vi "0. Using within CSM - Get Module Configuration.vi"() -> ()   [LabVIEW 2017]
uses:
  fc5fbf42-5c4f-4ff1-85ec-327809f3c502.vi
  a48643ac-d5d5-4d55-bcec-da4c3fe174fc.vi
  08dfc535-f17e-4bcc-abdf-94a82fd10ea0.vi
  <userlib>/_NEVSTOP/Communicable State Machine(CSM)/AdvanceAPI/CSM - Revert Arguments-Safe String.vi
  <userlib>/_NEVSTOP/Communicable State Machine(CSM)/AdvanceAPI/CSM - Make String Arguments Safe.vi
  <userlib>/_NEVSTOP/Communicable State Machine(CSM)/AdvanceAPI/CSM - Break Down Multiple States String.vi
  <userlib>/_NEVSTOP/Communicable State Machine(CSM)/AdvanceAPI/CSM - Compact Multiple States.vi
  <userlib>/_NEVSTOP/Communicable State Machine(CSM)/AdvanceAPI/CSM - Keywords.vi
  <userlib>/_NEVSTOP/Communicable State Machine(CSM)/_Shared/Trim Single-line Text.vi
  addons/API-String-Arugments-Support/_Support/Query Data as API String Arguments(variant).vi
  addons/API-String-Arugments-Support/_Support/Convert API String Arguments to Data(variant).vi
  <userlib>/_NEVSTOP/Communicable State Machine(CSM)/Communicable State Machine.lvlib
  addons/API-String-Arugments-Support/API String Arguments Support.lvlib
panel:
  out "string":string
  out "bool":bool
  out "dbl":dbl
  out "cluster.string2":string
  out "cluster.bool2":bool
  out "State History":string
  out "Configurations":string[](array[string])
  out "VI Path":path
  out "Core.Current VI Reference":variant
  out "Core.Current VI Reference":string="DoA"
  out "Settings":string="DoA"
  out "error out":errorcluster
  out "DataBool":string="DoA"
  out "DataString":string="DoA"
  out "Settings.Bool":string="DoA"
  out "Settings.String":string="DoA"
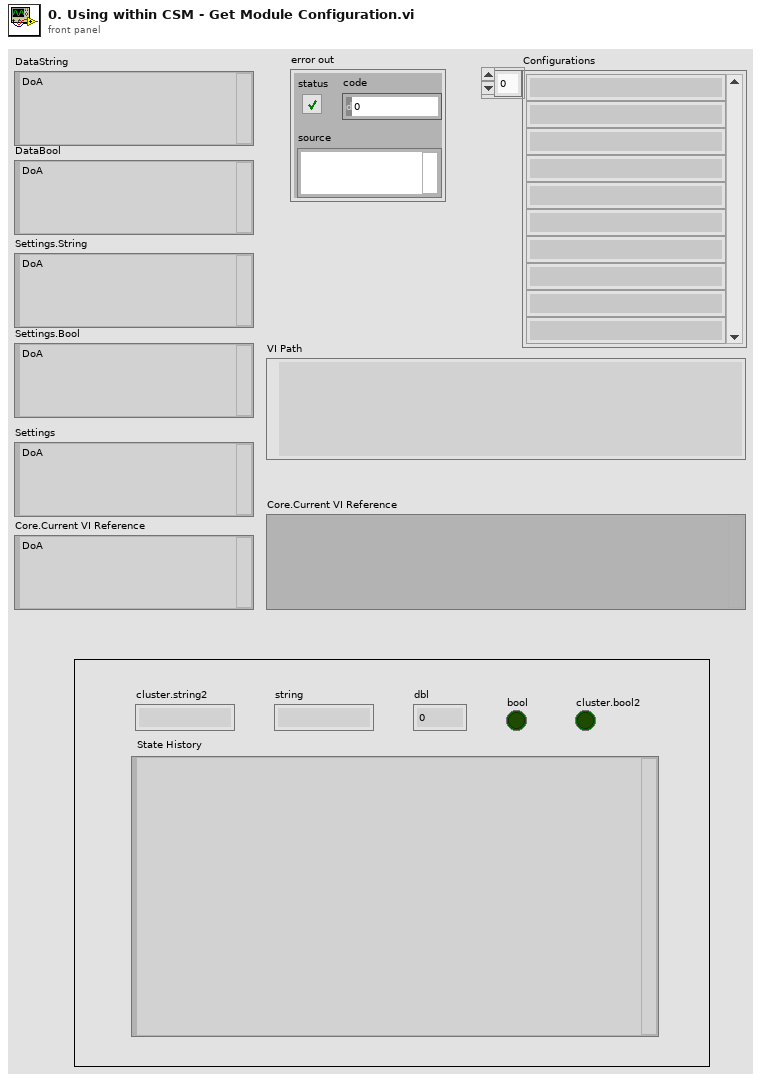
[diagram p1: front panel]
types:
  T1 = enum32{"Invalid", "Standard", "Closed", "Hidden", "Minimized", "Maximized"}
  T2 = enum32{"invalid app kind", "Development System", "Run Time System", "Student Edition", "Embedded LabVIEW", "Evaluation", "Custom"}
  T3 = typedef "Communicable State Machine.lvlib/_CSM_Response Source Message.ctl" = cluster{"‘State":string, "’Arguments":string, "’Error":errorcluster}
  T4 = cluster{"Current VI Reference":refnum<vi>, "Close Panel on Exit?":bool}
  T5 = cluster{"Core":cluster{"Current VI Reference":refnum<vi>, "Close Panel on Exit?":bool}, "DataBool":bool, "DataString":string, "Settings":cluster{"Bool":bool, "string":string}}
  T6 = cluster{"string":string, "bool":bool, "dbl":dbl, "cluster":cluster{"string2":string, "bool2":bool}}
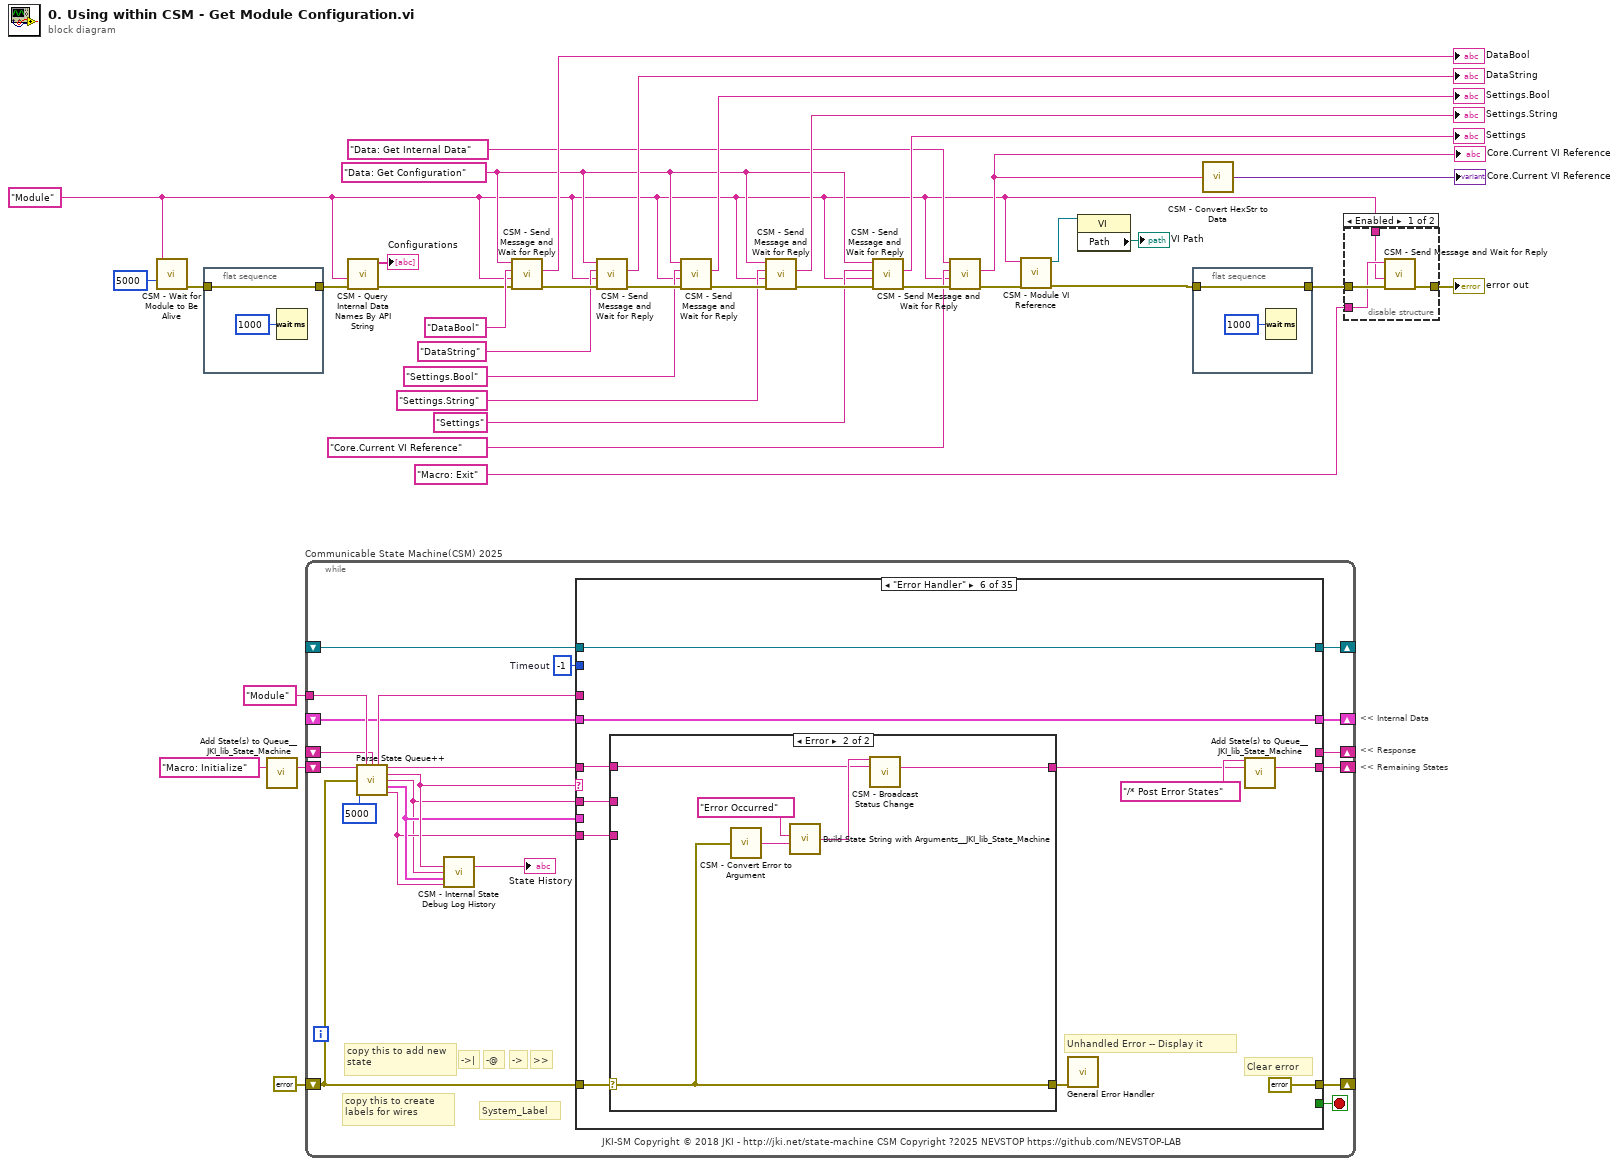
[diagram p0: block diagram]
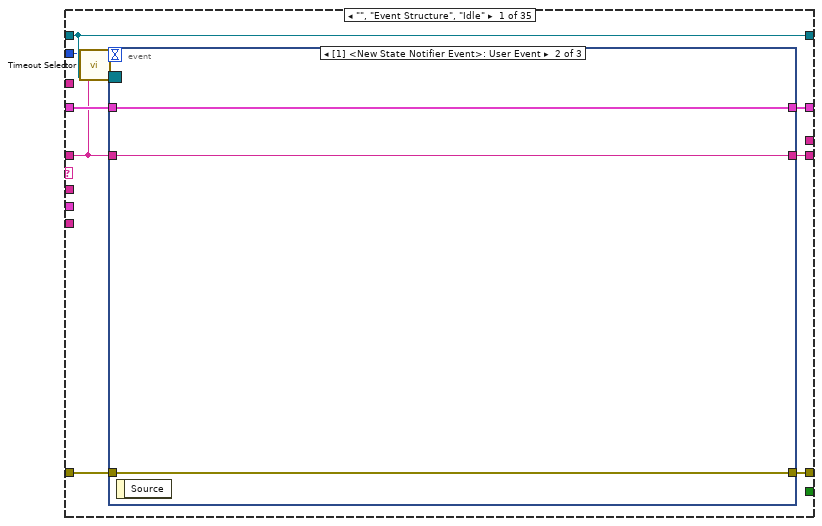
[diagram p2: hidden frame]
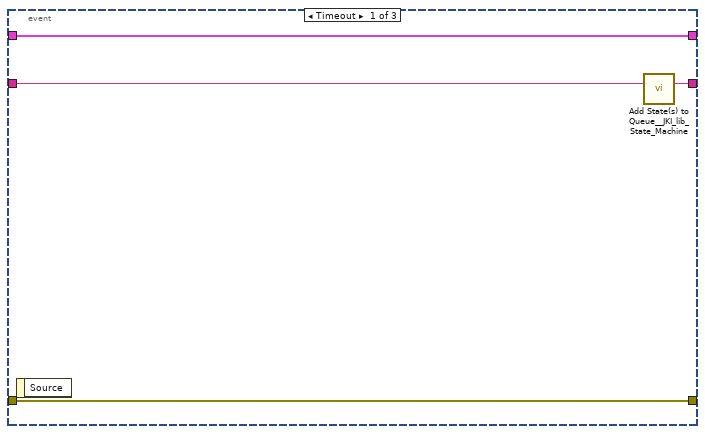
[diagram p3: hidden frame]
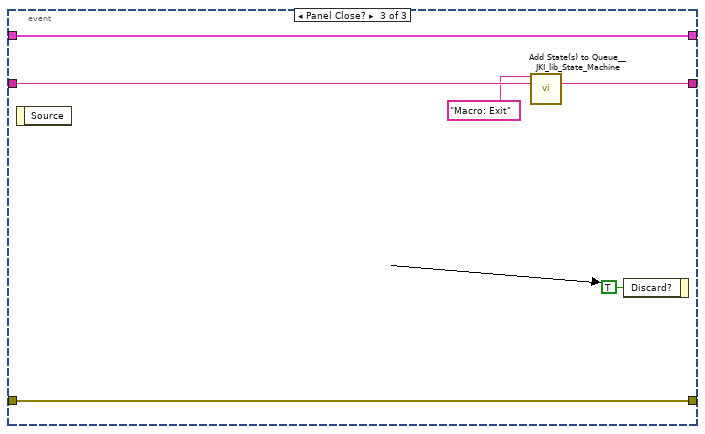
[diagram p4: hidden frame]
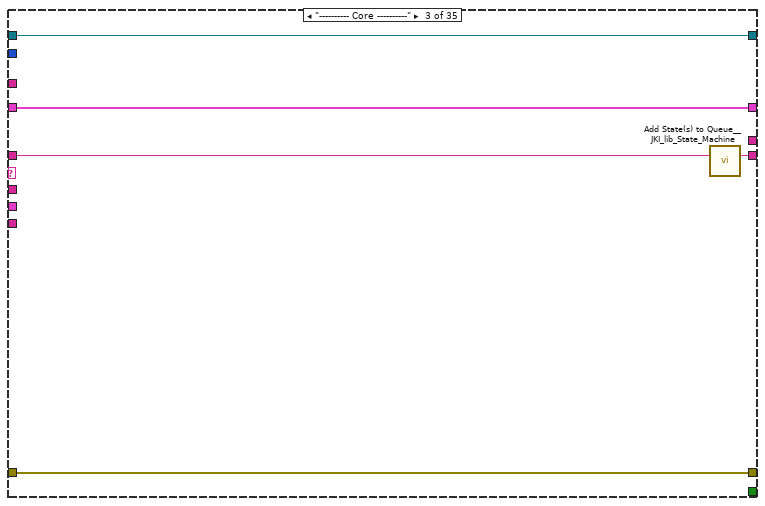
[diagram p6: hidden frame]
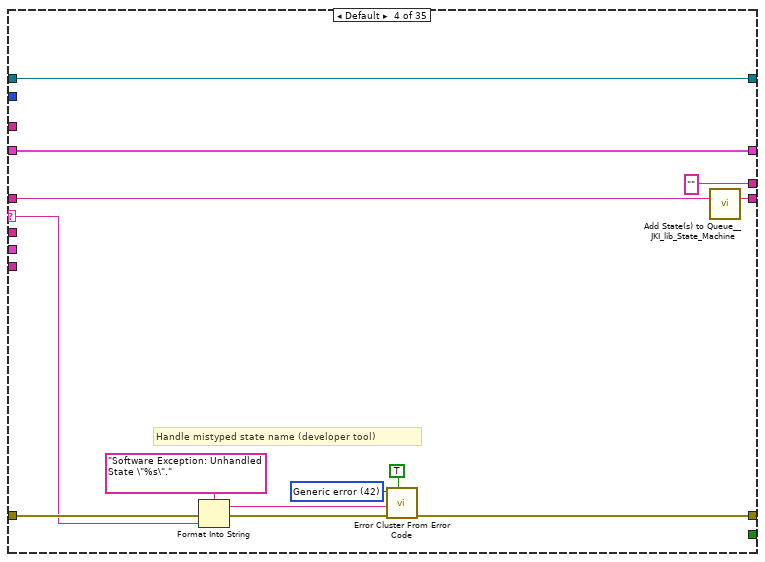
[diagram p7: hidden frame]
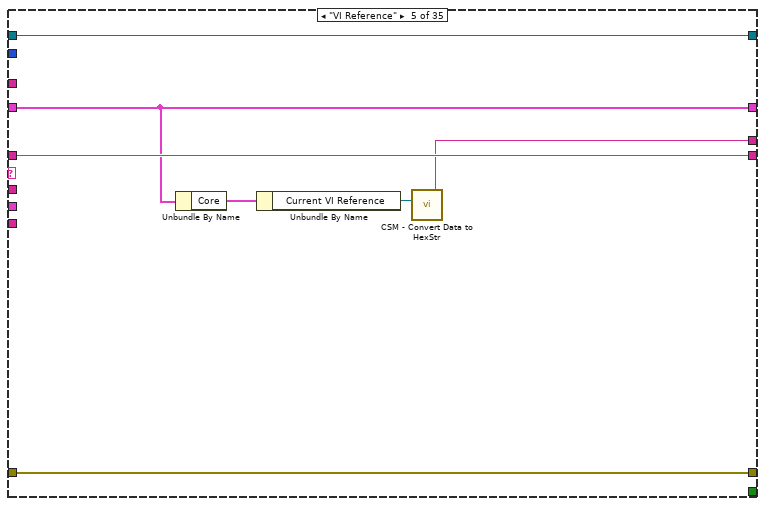
[diagram p8: hidden frame]
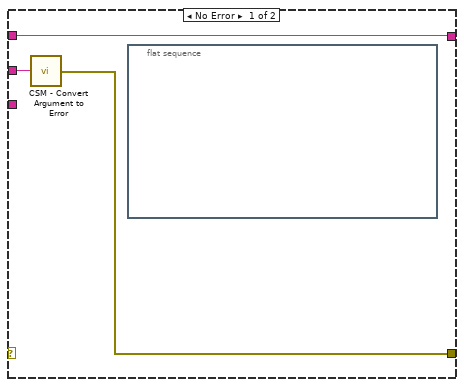
[diagram p9: hidden frame]
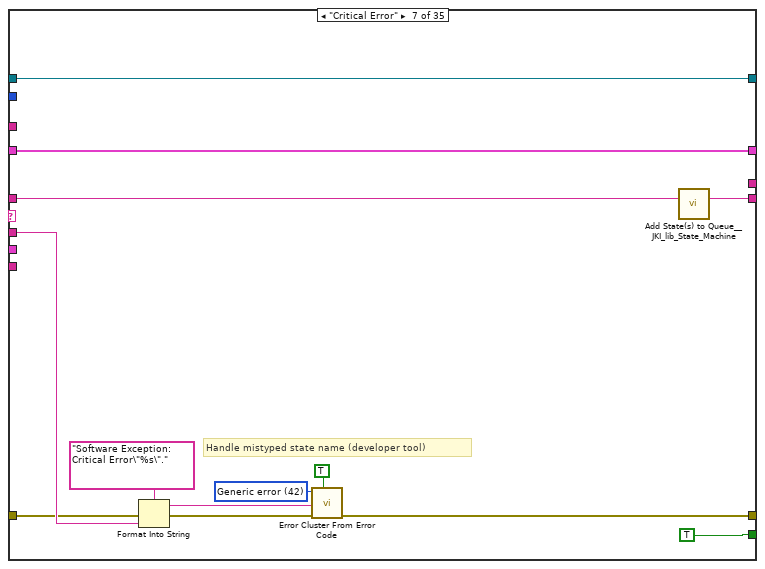
[diagram p10: hidden frame]
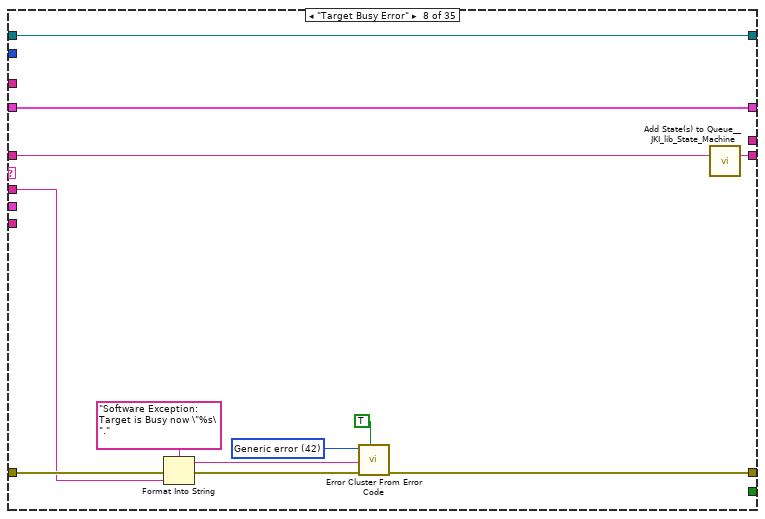
[diagram p11: hidden frame]
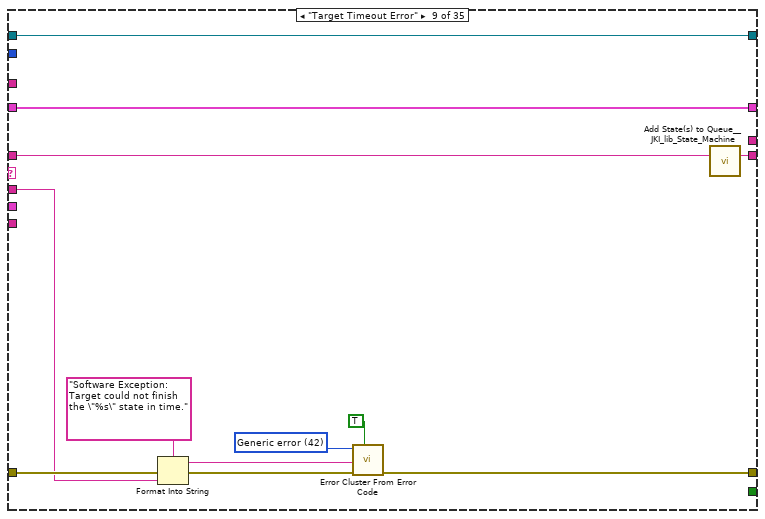
[diagram p12: hidden frame]
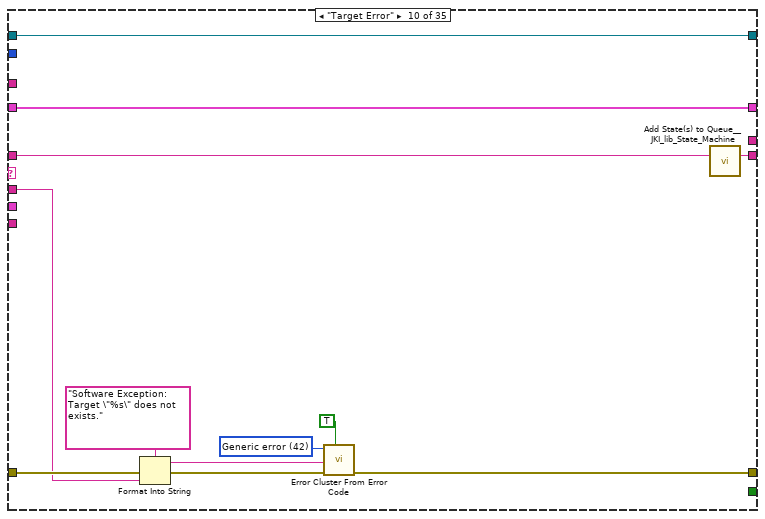
[diagram p13: hidden frame]
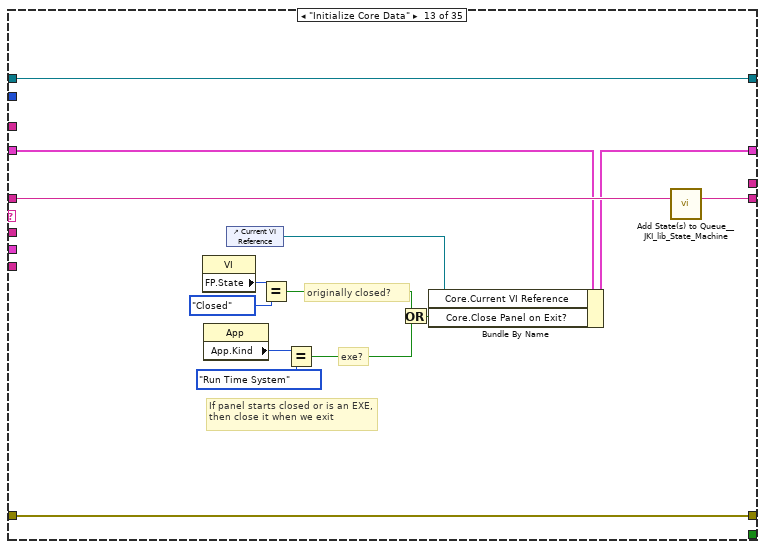
[diagram p16: hidden frame]
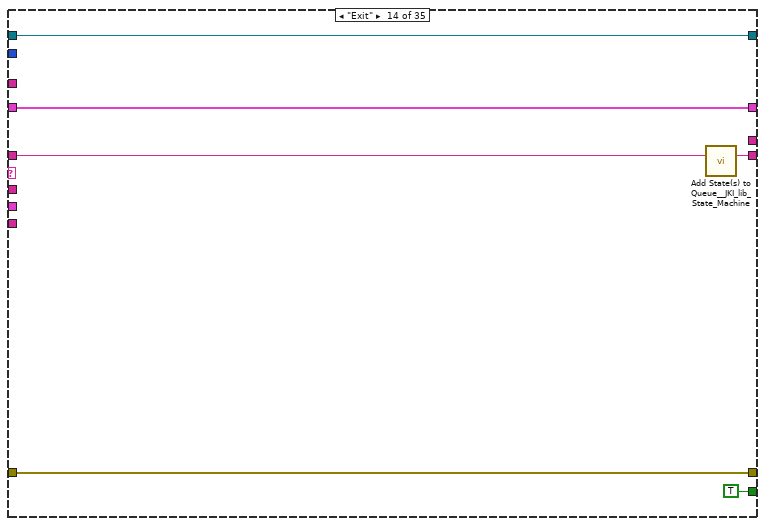
[diagram p17: hidden frame]
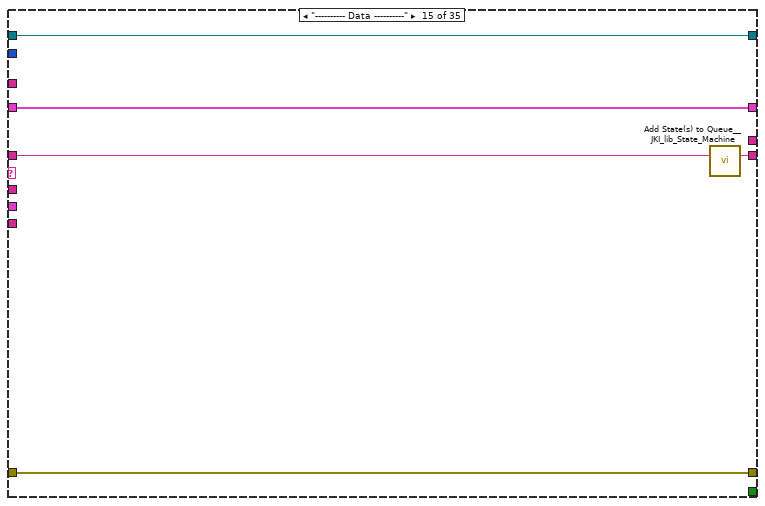
[diagram p18: hidden frame]
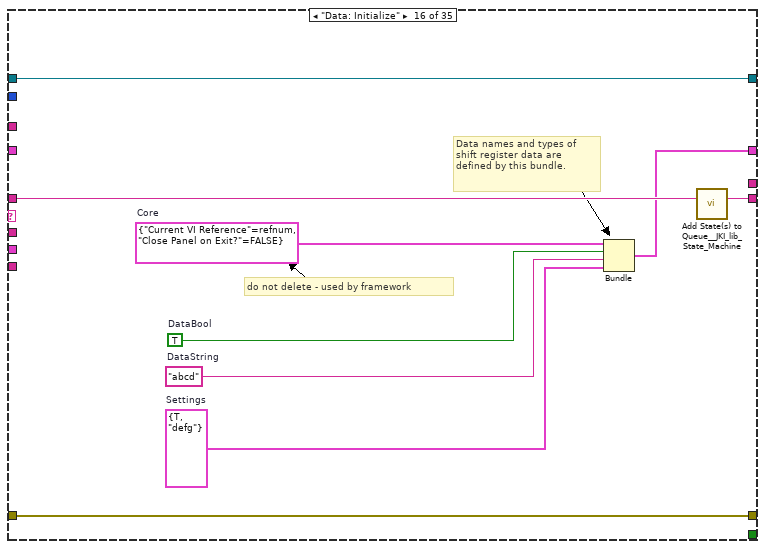
[diagram p19: hidden frame]
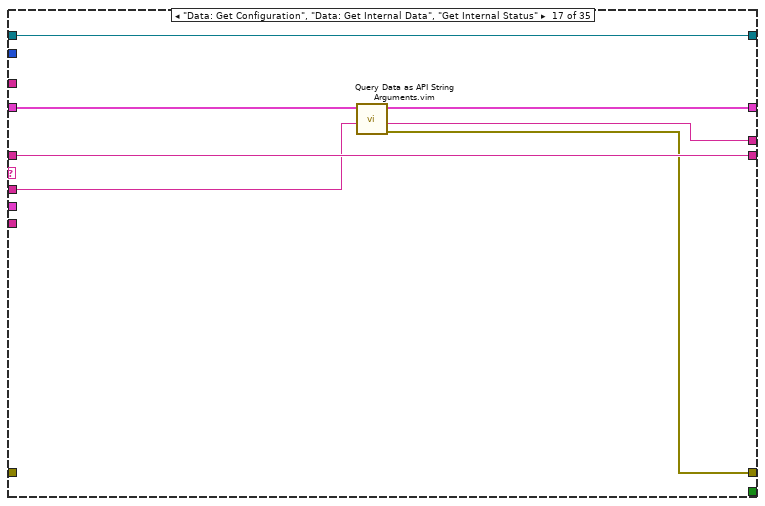
[diagram p20: hidden frame]
diagram:
  w22 = "Data: Get Configuration" ("Name(\"\" to use uuid)")
  w5 = "Module" ("Name(\"\" to use uuid)")
  # "<< Internal Data"
  # "<< Response"
  # "<< Remaining States"
  n1 = call <userlib>:"CSM - Wait for Module to Be Alive.vi"("CSM Name"=w5, "Wait (5000 ms)"=5000 ("Wait(5000ms)")) -> ("error out"=w7:errorcluster)  [unwired: 11 in, 2 out]
  n2 = flat-sequence {
    tunnel: [w39] -> w10
    tunnel: w7 -> [w39]
    frame #0 {
      n3 = Wait (ms)(milliseconds to wait=u32 1000) -> ()  [unwired: 1 out]
    }
  }
  n4 = call <vilib>:"Add State(s) to Queue__JKI_lib_State_Machine.vi"("State(s) in (\"\")"="Macro: Initialize") -> ("States Out"=w2:string)  [unwired: 14 in]
  n5 = while "Communicable State Machine(CSM) 2025" {
    shift-right: [w55] -> _
    shift-left: _ -> [w41]
    shift-right: [w58] -> _
    shift-left: errorcluster {"status"=FALSE, "code"=0, "source"=""} ("error") -> [w53]
    shift-right: [w57] -> _
    shift-left: w2 -> [w59]
    tunnel: "Module" ("Name(\"\" to use uuid)") -> [w48]
    shift-right: [w51] -> _
    shift-left: _ -> [w43]
    shift-right: [w50] -> _
    shift-left: _ -> [w49]
    stop <- w56 stop-if-true
    w54 = -1  # Timeout
    # "JKI-SM Copyright © 2018 JKI - http://jki.net/state-machine CSM Copyright ?2025 NEVSTOP https://github.com/NEVSTOP-LAB"
    # "->|"
    # "copy this to add new state"
    # ">>"
    # "->"
    # "-@"
    # "copy this to create labels for wires"
    # "System_Label"
    n6 = call <userlib>:"Parse State Queue++.vi"("State Queue"=w59, "Name (\"\" to Use UUID)"=w48, "Response Arguments"=w43, "Previous Error"=w53, "Response Timeout (-2 Use Global Settings)"=5000 ("Response Timeout(1000ms)")) -> ("Name Used"=w44:string, "Remaining States"=w60:string, "Current State"=w47:string, "Arguments"=w42:string, "Additional Information"=w46:T3, "Source CSM"=w45:string)  [unwired: 5 in]
    n7 = call <userlib>:"CSM - Internal State Debug Log History.vi"("State"=w47, "Arguments (\"\")"=w42, ">> Response Source Message >>"=w46, "Source (\"\")"=w45) -> ("Debug Log"=→"State History":string)  [unwired: 11 in]
    n8 = case shown="\"Error Handler\"" w47 {
      selector: w47 -> [_ _ _ w94 _ _ _ _ _ _ _ _ _ _ _ _ _ _ _ _ _ _ _ _ _ _ _ _ _ _ _ _ _ _ _]
      tunnel: w60 -> [w61 w86 w91 w98 w110 w115 w143 w146 w163 w175 w183 w187 w202 w208 w213 w222 w229 w235 w242 w247 w254 w258 w264 w269 w276 w292 w362 w368 w379 w382 w395 w398 w404 w409 w414]
      tunnel: w42 -> [_ _ _ _ _ w113 w136 w148 w159 w171 _ _ _ _ _ _ w224 w233 _ _ _ _ _ _ w271 w286 _ _ _ _ w391 _ _ _ _]
      tunnel: w41 -> [w68 w85 w88 w96 w106 w121 w144 w150 w161 w173 w182 w186 w195 w206 w210 _ w227 w232 w237 w244 w253 w257 w261 w267 w274 w288 w359 w365 w376 w381 w394 w397 w401 w406 w411]
      tunnel: [w67 w84 w89 w100 w111 errorcluster {"status"=FALSE, "code"=0, "source"=""} ("error out") w132 w145 w157 w169 w184 w188 w199 w205 w211 w219 w225 w230 w238 w245 w248 w256 w262 w266 w272 w289 w360 w366 w377 w383 w384 w399 w402 w407 w412] -> w58
      tunnel: w53 -> [w66 w84 w89 w99 w111 w119 w133 w152 w164 w176 w184 w188 w199 w205 w211 w219 _ _ w239 w245 _ w259 w262 w266 w273 w290 w360 w366 w377 w383 _ w399 w402 w407 w412]
      tunnel: [w69 w86 w90 w97 w110 w117 w142 w151 w162 w174 w183 w187 w201 w207 w212 w221 w229 w235 w241 w246 w254 w258 w263 w268 w275 w291 w361 w367 w378 w382 w395 w398 w403 w408 w413] -> w57
      tunnel: [_ _ _ _ _ _ TRUE _ _ _ _ _ _ TRUE _ _ _ _ _ _ _ _ _ _ _ _ _ _ _ _ _ _ _ _ _] -> w56
      tunnel: [w65 w85 w88 w96 w106 w121 w144 w150 w161 w173 w182 w186 w200 w206 w210 w220 w223 w231 w237 w244 w253 w257 w261 w267 w274 w288 w359 w365 w376 w381 w394 w397 w401 w406 w411] -> w55
      tunnel: w54 -> [w63 _ _ _ _ _ _ _ _ _ _ _ _ _ _ _ _ _ _ _ _ _ _ _ _ _ _ _ _ _ _ _ _ _ _]
      tunnel: w45 -> [_ _ _ _ _ w112 _ _ _ _ _ _ _ _ _ _ _ _ _ _ _ _ _ _ _ _ _ _ _ _ _ _ _ _ _]
      tunnel: w46 -> [_ _ _ _ _ _ _ _ _ _ _ _ _ _ _ _ _ _ _ _ _ _ _ _ _ _ _ _ _ _ _ _ _ _ _]
      tunnel: [_ _ _ "" w105 _ _ _ _ _ _ _ _ _ _ _ w226 _ _ _ _ _ _ _ _ _ _ _ _ _ _ _ _ _ _] -> w51
      tunnel: [w64 w83 w87 w92 w109 w120 w134 w147 w158 w170 w181 w185 w189 w203 w209 w215 w228 w234 w236 w243 w252 w255 w260 w265 w270 w285 w358 w363 w369 w380 w393 w396 w400 w405 w410] -> w50
      tunnel: w49 -> [w64 w83 w87 w92 w109 w120 w134 w147 w158 w170 w181 w185 w189 w203 w209 w215 w228 w234 w236 w243 _ w255 w260 w265 w270 w285 w358 w363 w369 w380 w393 w396 w400 w405 w410]
      tunnel: w44 -> [_ _ _ _ _ _ _ _ _ _ _ _ _ _ _ _ _ _ _ _ w251 _ _ _ _ _ _ _ _ _ _ _ _ _ _]
      frame "", "Event Structure", "Idle" {
        n9 = call <userlib>:"Timeout Selector.vi"("Remaining States"=w61, "Timeout Expected"=w63) -> ("Timeout"=w62:i32)  [unwired: 5 in]
        n10 = event shown="[1] <New State Notifier Event>: User Event" {
          selector: w64 -> [_ _ _]
          dyn-events: _ -> [_ _ _]
          timeout: w62 -> [_ _ _]
          tunnel: w61 -> [w73 w75 w82]
          tunnel: [w72 w75 w81] -> w69
          tunnel: w68 -> [w70 w76 w79]
          tunnel: [w71 w74 w80] -> w67
          tunnel: w66 -> [w71 w74 w80]
          tunnel: [w70 w76 w79] -> w65
          event Timeout {
            n11 = event-data() -> ()  [unwired: 1 in, 1 out]
            n12 = call <vilib>:"Add State(s) to Queue__JKI_lib_State_Machine.vi"("State(s) in (\"\")"=w73) -> ("States Out"=w72:string)  [unwired: 14 in]
          }
          event User Event {
            n13 = event-data() -> ()  [unwired: 1 in, 1 out]
          }
          event Panel Close? {
            n14 = event-data() -> ()  [unwired: 1 in, 1 out]
            n15 = call <vilib>:"Add State(s) to Queue__JKI_lib_State_Machine.vi"("State(s) in Front (\"\")"="Macro: Exit", "State(s) in (\"\")"=w82) -> ("States Out"=w81:string)  [unwired: 13 in]
            n16 = event-data("Discard?"=TRUE) -> ()  [unwired: 1 in, 1 out]
          }
        }
      }
      frame "CSM Documentation" {
        # "CSM Documentation"
      }
      frame "---------- Core ----------" {
        n17 = call <vilib>:"Add State(s) to Queue__JKI_lib_State_Machine.vi"("State(s) in (\"\")"=w91) -> ("States Out"=w90:string)  [unwired: 14 in]
      }
      frame Default {
        w103 = 42 items=["No error", "Argument error", "Memory is full", "Out of zone", "End of file", "File already open", "Generic file I/O error", "File not found", "File permission error", "Disk is full", "Duplicate path", "Too many files open", "System feature not enabled", "Resource file not found", "Cannot add resource", "Resource not found", "Image not found", "Image memory error", "Pen does not exist", "Config type invalid", "Config token not found", "Config parse error", "Config memory error", "Bad external code format", "Bad external code offset", "External code not present", "Null window", "Destroy window error", "Null menu", "Print aborted", "Bad print record", "Print driver error", "Windows error during printing", "Memory error during printing", "Print dialog error", "Generic print error", "Invalid device refnum", "Device not found", "Device parameter error", "Device unit error", "Cannot open device", "Device call aborted", "Generic error", "Cancelled by user", "Object ID too low", "Object ID too high", "Object not in heap", "Unknown heap", "Unknown object (invalid DefProc)", "Unknown object (DefProc not in table)", "Message out of range", "Invalid (null) method", "Unknown message", "Manager call not supported", "Bad address", "Network operation in progress", "Network operation timed out", "Connection is busy", "Network attribute not supported", "Network error", "Address in use", "System out of memory", "Connection aborted", "Connection refused", "Not connected", "Already connected", "Connection closed", "Initialization error (interapplication manager)", "Bad occurrence", "Wait on unbound occurrence handler", "Occurrence queue overflow", "Datalog type conflict", "Unused", "Unrecognized type (interapplication manager)", "Memory corrupt", "Failed to make temporary DLL", "Old CIN version", "Drag socket not found", "Failed to load drop-object", "Failed to register OLE object", "Failed to release OLE object", "Format specifier type mismatch", "Unknown format specifier", "Too few format specifiers", "Too many format specifiers", "Scan failed", "Newer CIN version", "Error converting to variant", "Runtime menu error", "Password tampered", "Variant attribute not found", "Incompatible variant data type", "Event data is not available", "Event Store is not present", "Occurrence is not found", "Event Queue is not created", "Event info is not available", "Refnum passed is NULL", "Error retrieving Class GUID", "Error retrieving CoClass GUID", "Error retrieving TypeLib GUID.", "Bad built application magic bytes.", "Specific driver is different from the specific driver associated with the Logical Name.", "There is no session opened to the class driver.", "Max Error", "MAX - Error with config objects", "MAX - Error loading configuration", "MAX - Group not supported"]
        # "Handle mistyped state name (developer tool)"
        n18 = Format Into String(format string="Software Exception: Unhandled State \"%s\"." ("message"), error in=w99, w94) -> (resulting string=w102:string, error out=w101:errorcluster)  [unwired: 1 in]
        n19 = call <vilib>:"Error Cluster From Error Code.vi"("show call chain? (False)"=TRUE, "error in (no error)"=w101, "error message (\"\")"=w102, "error code (0)"=w103) -> ("error out"=w100:errorcluster)  [unwired: 5 in]
        n20 = call <vilib>:"Add State(s) to Queue__JKI_lib_State_Machine.vi"("State(s) in (\"\")"=w98) -> ("States Out"=w97:string)  [unwired: 14 in]
      }
      frame "VI Reference" {
        n21 = Unbundle By Name(w106) -> ("Core"=w108:T4)
        n22 = Unbundle By Name(w108) -> ("Current VI Reference"=w107:refnum<vi>)
        n23 = call <userlib>:"CSM - Convert Data to HexStr.vi"("Variant"=w107) -> ("HEX String (0-9,A-F)"=w105:string)  [unwired: 8 in]
      }
      frame "Error Handler" {
        # "Unhandled Error -- Display it"
        # "Clear error"
        n24 = case shown="Error" w119 {
          selector: w119 -> [_ w126]
          tunnel: [w124 w128] -> w116
          tunnel: w115 -> [w124 w127]
          tunnel: [w123 w126] -> w114
          tunnel: w113 -> [w125 _]
          tunnel: w112 -> [_ _]
          frame No Error {
            n25 = call <userlib>:"CSM - Convert Argument to Error.vi"("Argument"=w125) -> ("Error"=w123:errorcluster)  [unwired: 4 in]
            n26 = flat-sequence {
              frame #0 {
              }
            }
          }
          frame Error {
            n27 = call <userlib>:"CSM - Convert Error to Argument.vi"("Error"=w126) -> ("Argument"=w130:string)  [unwired: 4 in]
            n28 = call <vilib>:"Build State String with Arguments__JKI_lib_State_Machine.vi"("Arguments (\"\")"=w130, "State"="Error Occurred" ("Status with Arguments")) -> ("State with Arguments"=w129:string)  [unwired: 4 in]
            n29 = call <userlib>:"CSM - Broadcast Status Change.vi"("Status With Arguments"=w129, "State Queue"=w127) -> ("Remaining States"=w128:string)  [unwired: 13 in]
          }
        }
        n30 = call <vilib>:"General Error Handler.vi"("error in (no error)"=w114) -> ()  [unwired: 10 in, 5 out]
        n31 = call <vilib>:"Add State(s) to Queue__JKI_lib_State_Machine.vi"("State(s) in Front (\"\")"="/* Post Error States", "State(s) in (\"\")"=w116) -> ("States Out"=w117:string)  [unwired: 13 in]
      }
      frame "Critical Error" {
        w140 = 42 items=["No error", "Argument error", "Memory is full", "Out of zone", "End of file", "File already open", "Generic file I/O error", "File not found", "File permission error", "Disk is full", "Duplicate path", "Too many files open", "System feature not enabled", "Resource file not found", "Cannot add resource", "Resource not found", "Image not found", "Image memory error", "Pen does not exist", "Config type invalid", "Config token not found", "Config parse error", "Config memory error", "Bad external code format", "Bad external code offset", "External code not present", "Null window", "Destroy window error", "Null menu", "Print aborted", "Bad print record", "Print driver error", "Windows error during printing", "Memory error during printing", "Print dialog error", "Generic print error", "Invalid device refnum", "Device not found", "Device parameter error", "Device unit error", "Cannot open device", "Device call aborted", "Generic error", "Cancelled by user", "Object ID too low", "Object ID too high", "Object not in heap", "Unknown heap", "Unknown object (invalid DefProc)", "Unknown object (DefProc not in table)", "Message out of range", "Invalid (null) method", "Unknown message", "Manager call not supported", "Bad address", "Network operation in progress", "Network operation timed out", "Connection is busy", "Network attribute not supported", "Network error", "Address in use", "System out of memory", "Connection aborted", "Connection refused", "Not connected", "Already connected", "Connection closed", "Initialization error (interapplication manager)", "Bad occurrence", "Wait on unbound occurrence handler", "Occurrence queue overflow", "Datalog type conflict", "Unused", "Unrecognized type (interapplication manager)", "Memory corrupt", "Failed to make temporary DLL", "Old CIN version", "Drag socket not found", "Failed to load drop-object", "Failed to register OLE object", "Failed to release OLE object", "Format specifier type mismatch", "Unknown format specifier", "Too few format specifiers", "Too many format specifiers", "Scan failed", "Newer CIN version", "Error converting to variant", "Runtime menu error", "Password tampered", "Variant attribute not found", "Incompatible variant data type", "Event data is not available", "Event Store is not present", "Occurrence is not found", "Event Queue is not created", "Event info is not available", "Refnum passed is NULL", "Error retrieving Class GUID", "Error retrieving CoClass GUID", "Error retrieving TypeLib GUID.", "Bad built application magic bytes.", "Specific driver is different from the specific driver associated with the Logical Name.", "There is no session opened to the class driver.", "Max Error", "MAX - Error with config objects", "MAX - Error loading configuration", "MAX - Group not supported"]
        # "Handle mistyped state name (developer tool)"
        n32 = Format Into String(format string="Software Exception: Critical Error\"%s\"." ("message"), error in=w133, w136) -> (resulting string=w139:string, error out=w138:errorcluster)  [unwired: 1 in]
        n33 = call <vilib>:"Error Cluster From Error Code.vi"("show call chain? (False)"=TRUE, "error in (no error)"=w138, "error message (\"\")"=w139, "error code (0)"=w140) -> ("error out"=w132:errorcluster)  [unwired: 5 in]
        n34 = call <vilib>:"Add State(s) to Queue__JKI_lib_State_Machine.vi"("State(s) in (\"\")"=w143) -> ("States Out"=w142:string)  [unwired: 14 in]
      }
      frame "Target Busy Error" {
        w155 = 42 items=["No error", "Argument error", "Memory is full", "Out of zone", "End of file", "File already open", "Generic file I/O error", "File not found", "File permission error", "Disk is full", "Duplicate path", "Too many files open", "System feature not enabled", "Resource file not found", "Cannot add resource", "Resource not found", "Image not found", "Image memory error", "Pen does not exist", "Config type invalid", "Config token not found", "Config parse error", "Config memory error", "Bad external code format", "Bad external code offset", "External code not present", "Null window", "Destroy window error", "Null menu", "Print aborted", "Bad print record", "Print driver error", "Windows error during printing", "Memory error during printing", "Print dialog error", "Generic print error", "Invalid device refnum", "Device not found", "Device parameter error", "Device unit error", "Cannot open device", "Device call aborted", "Generic error", "Cancelled by user", "Object ID too low", "Object ID too high", "Object not in heap", "Unknown heap", "Unknown object (invalid DefProc)", "Unknown object (DefProc not in table)", "Message out of range", "Invalid (null) method", "Unknown message", "Manager call not supported", "Bad address", "Network operation in progress", "Network operation timed out", "Connection is busy", "Network attribute not supported", "Network error", "Address in use", "System out of memory", "Connection aborted", "Connection refused", "Not connected", "Already connected", "Connection closed", "Initialization error (interapplication manager)", "Bad occurrence", "Wait on unbound occurrence handler", "Occurrence queue overflow", "Datalog type conflict", "Unused", "Unrecognized type (interapplication manager)", "Memory corrupt", "Failed to make temporary DLL", "Old CIN version", "Drag socket not found", "Failed to load drop-object", "Failed to register OLE object", "Failed to release OLE object", "Format specifier type mismatch", "Unknown format specifier", "Too few format specifiers", "Too many format specifiers", "Scan failed", "Newer CIN version", "Error converting to variant", "Runtime menu error", "Password tampered", "Variant attribute not found", "Incompatible variant data type", "Event data is not available", "Event Store is not present", "Occurrence is not found", "Event Queue is not created", "Event info is not available", "Refnum passed is NULL", "Error retrieving Class GUID", "Error retrieving CoClass GUID", "Error retrieving TypeLib GUID.", "Bad built application magic bytes.", "Specific driver is different from the specific driver associated with the Logical Name.", "There is no session opened to the class driver.", "Max Error", "MAX - Error with config objects", "MAX - Error loading configuration", "MAX - Group not supported"]
        n35 = Format Into String(format string="Software Exception: Target is Busy now \"%s\"." ("message"), error in=w152, w148) -> (resulting string=w154:string, error out=w153:errorcluster)  [unwired: 1 in]
        n36 = call <vilib>:"Error Cluster From Error Code.vi"("show call chain? (False)"=TRUE, "error in (no error)"=w153, "error message (\"\")"=w154, "error code (0)"=w155) -> ("error out"=w145:errorcluster)  [unwired: 5 in]
        n37 = call <vilib>:"Add State(s) to Queue__JKI_lib_State_Machine.vi"("State(s) in (\"\")"=w146) -> ("States Out"=w151:string)  [unwired: 14 in]
      }
      frame "Target Timeout Error" {
        w167 = 42 items=["No error", "Argument error", "Memory is full", "Out of zone", "End of file", "File already open", "Generic file I/O error", "File not found", "File permission error", "Disk is full", "Duplicate path", "Too many files open", "System feature not enabled", "Resource file not found", "Cannot add resource", "Resource not found", "Image not found", "Image memory error", "Pen does not exist", "Config type invalid", "Config token not found", "Config parse error", "Config memory error", "Bad external code format", "Bad external code offset", "External code not present", "Null window", "Destroy window error", "Null menu", "Print aborted", "Bad print record", "Print driver error", "Windows error during printing", "Memory error during printing", "Print dialog error", "Generic print error", "Invalid device refnum", "Device not found", "Device parameter error", "Device unit error", "Cannot open device", "Device call aborted", "Generic error", "Cancelled by user", "Object ID too low", "Object ID too high", "Object not in heap", "Unknown heap", "Unknown object (invalid DefProc)", "Unknown object (DefProc not in table)", "Message out of range", "Invalid (null) method", "Unknown message", "Manager call not supported", "Bad address", "Network operation in progress", "Network operation timed out", "Connection is busy", "Network attribute not supported", "Network error", "Address in use", "System out of memory", "Connection aborted", "Connection refused", "Not connected", "Already connected", "Connection closed", "Initialization error (interapplication manager)", "Bad occurrence", "Wait on unbound occurrence handler", "Occurrence queue overflow", "Datalog type conflict", "Unused", "Unrecognized type (interapplication manager)", "Memory corrupt", "Failed to make temporary DLL", "Old CIN version", "Drag socket not found", "Failed to load drop-object", "Failed to register OLE object", "Failed to release OLE object", "Format specifier type mismatch", "Unknown format specifier", "Too few format specifiers", "Too many format specifiers", "Scan failed", "Newer CIN version", "Error converting to variant", "Runtime menu error", "Password tampered", "Variant attribute not found", "Incompatible variant data type", "Event data is not available", "Event Store is not present", "Occurrence is not found", "Event Queue is not created", "Event info is not available", "Refnum passed is NULL", "Error retrieving Class GUID", "Error retrieving CoClass GUID", "Error retrieving TypeLib GUID.", "Bad built application magic bytes.", "Specific driver is different from the specific driver associated with the Logical Name.", "There is no session opened to the class driver.", "Max Error", "MAX - Error with config objects", "MAX - Error loading configuration", "MAX - Group not supported"]
        n38 = Format Into String(format string="Software Exception: Target could not finish the \"%s\" state in time." ("message"), error in=w164, w159) -> (resulting string=w166:string, error out=w165:errorcluster)  [unwired: 1 in]
        n39 = call <vilib>:"Error Cluster From Error Code.vi"("show call chain? (False)"=TRUE, "error in (no error)"=w165, "error message (\"\")"=w166, "error code (0)"=w167) -> ("error out"=w157:errorcluster)  [unwired: 5 in]
        n40 = call <vilib>:"Add State(s) to Queue__JKI_lib_State_Machine.vi"("State(s) in (\"\")"=w163) -> ("States Out"=w162:string)  [unwired: 14 in]
      }
      frame "Target Error" {
        w179 = 42 items=["No error", "Argument error", "Memory is full", "Out of zone", "End of file", "File already open", "Generic file I/O error", "File not found", "File permission error", "Disk is full", "Duplicate path", "Too many files open", "System feature not enabled", "Resource file not found", "Cannot add resource", "Resource not found", "Image not found", "Image memory error", "Pen does not exist", "Config type invalid", "Config token not found", "Config parse error", "Config memory error", "Bad external code format", "Bad external code offset", "External code not present", "Null window", "Destroy window error", "Null menu", "Print aborted", "Bad print record", "Print driver error", "Windows error during printing", "Memory error during printing", "Print dialog error", "Generic print error", "Invalid device refnum", "Device not found", "Device parameter error", "Device unit error", "Cannot open device", "Device call aborted", "Generic error", "Cancelled by user", "Object ID too low", "Object ID too high", "Object not in heap", "Unknown heap", "Unknown object (invalid DefProc)", "Unknown object (DefProc not in table)", "Message out of range", "Invalid (null) method", "Unknown message", "Manager call not supported", "Bad address", "Network operation in progress", "Network operation timed out", "Connection is busy", "Network attribute not supported", "Network error", "Address in use", "System out of memory", "Connection aborted", "Connection refused", "Not connected", "Already connected", "Connection closed", "Initialization error (interapplication manager)", "Bad occurrence", "Wait on unbound occurrence handler", "Occurrence queue overflow", "Datalog type conflict", "Unused", "Unrecognized type (interapplication manager)", "Memory corrupt", "Failed to make temporary DLL", "Old CIN version", "Drag socket not found", "Failed to load drop-object", "Failed to register OLE object", "Failed to release OLE object", "Format specifier type mismatch", "Unknown format specifier", "Too few format specifiers", "Too many format specifiers", "Scan failed", "Newer CIN version", "Error converting to variant", "Runtime menu error", "Password tampered", "Variant attribute not found", "Incompatible variant data type", "Event data is not available", "Event Store is not present", "Occurrence is not found", "Event Queue is not created", "Event info is not available", "Refnum passed is NULL", "Error retrieving Class GUID", "Error retrieving CoClass GUID", "Error retrieving TypeLib GUID.", "Bad built application magic bytes.", "Specific driver is different from the specific driver associated with the Logical Name.", "There is no session opened to the class driver.", "Max Error", "MAX - Error with config objects", "MAX - Error loading configuration", "MAX - Group not supported"]
        n41 = Format Into String(format string="Software Exception: Target \"%s\" does not exists." ("message"), error in=w176, w171) -> (resulting string=w178:string, error out=w177:errorcluster)  [unwired: 1 in]
        n42 = call <vilib>:"Error Cluster From Error Code.vi"("show call chain? (False)"=TRUE, "error in (no error)"=w177, "error message (\"\")"=w178, "error code (0)"=w179) -> ("error out"=w169:errorcluster)  [unwired: 5 in]
        n43 = call <vilib>:"Add State(s) to Queue__JKI_lib_State_Machine.vi"("State(s) in (\"\")"=w175) -> ("States Out"=w174:string)  [unwired: 14 in]
      }
      frame "Async Response", "Response" {
      }
      frame "Async Message Posted" {
      }
      frame "Initialize Core Data" {
        # "originally closed?"
        # "exe?"
        # "If panel starts closed or is an EXE, then close it when we exit"
        n44 = property class="VI"() -> ("FP.State"=w192:T1)  [unwired: 2 in, 2 out]
        n45 = property class="App"() -> ("App.Kind"=w198:T2)  [unwired: 2 in, 2 out]
        n46 = control-ref of="Current VI Reference"() -> (w193:refnum<vi>)
        n47 = Equal?(x=w192, y=T1."Closed" ("Front Panel Window:State")) -> (x = y?=w190:bool)
        n48 = Equal?(x=w198, y=T2."Run Time System" ("Application:Kind")) -> (x = y?=w196:bool)
        n49 = Or(x=w190, y=w196) -> (x .or. y?=w194:bool)
        n50 = Bundle By Name(cluster=w195, "Core.Current VI Reference"=w193, "Core.Close Panel on Exit?"=w194) -> (w200:T5)
        n51 = call <vilib>:"Add State(s) to Queue__JKI_lib_State_Machine.vi"("State(s) in (\"\")"=w202) -> ("States Out"=w201:string)  [unwired: 14 in]
      }
      frame "Exit" {
        n52 = call <vilib>:"Add State(s) to Queue__JKI_lib_State_Machine.vi"("State(s) in (\"\")"=w208) -> ("States Out"=w207:string)  [unwired: 14 in]
      }
      frame "---------- Data ----------" {
        n53 = call <vilib>:"Add State(s) to Queue__JKI_lib_State_Machine.vi"("State(s) in (\"\")"=w213) -> ("States Out"=w212:string)  [unwired: 14 in]
      }
      frame "Data: Initialize" {
        w214 = cluster{"Bool":bool, "string":string} {"Bool"=TRUE, "string"="defg"}  # Settings
        w216 = T4 {"Current VI Reference"=refnum, "Close Panel on Exit?"=FALSE}  # Core
        w218 = TRUE  # DataBool
        w217 = "abcd"  # DataString
        # "do not delete - used by framework"
        # "Data names and types of shift register data are defined by this bundle."
        n54 = Bundle("Core"=w216, "DataBool"=w218, "DataString"=w217, "Settings"=w214) -> (w220:T5)  [unwired: 1 in]
        n55 = call <vilib>:"Add State(s) to Queue__JKI_lib_State_Machine.vi"("State(s) in (\"\")"=w222) -> ("States Out"=w221:string)  [unwired: 14 in]
      }
      frame "Data: Get Configuration", "Data: Get Internal Data", "Get Internal Status" {
        n56 = call "Query Data as API String Arguments.vim"("Name"=w224, "Cluster Data"=w227) -> ("error"=w225:errorcluster, "API String"=w226:string, "Cluster Data (dup)"=w223:T5)  [unwired: 7 in]
      }
      frame "Data: Set Configuration" {
        n57 = call "Convert API String Arguments to Data.vim"("Reference Type"=w232, "API String"=w233) -> ("error out"=w230:errorcluster, "Data"=w231:T5)  [unwired: 6 in]
      }
      frame "Data: Cleanup" {
        n58 = Unbundle By Name(w237) -> ("Core.Current VI Reference"=w240:refnum<vi>)
        n59 = Close Reference(reference=w240, error in (no error)=w239) -> (error out=w238:errorcluster)
        n60 = call <vilib>:"Add State(s) to Queue__JKI_lib_State_Machine.vi"("State(s) in (\"\")"=w242) -> ("States Out"=w241:string)  [unwired: 14 in]
      }
      frame "---------- Events ----------" {
        n61 = call <vilib>:"Add State(s) to Queue__JKI_lib_State_Machine.vi"("State(s) in (\"\")"=w247) -> ("States Out"=w246:string)  [unwired: 14 in]
      }
      frame "Events: Register" {
        n62 = call <userlib>:"CSM - Get New State Notifier Event.vi"("Name (\"\" to Use UUID)"=w251) -> ("error out"=w249:errorcluster, "New State Notifier Event"=w250:refnum<user-event>)  [unwired: 9 in]
        n63 = register-events(error in=w249, w250) -> (reference out=w252:refnum<event-registration>, error out=w248:errorcluster)  [unwired: 1 in]
      }
      frame "Events: Unregister" {
        n64 = Unregister For Events(event registration refnum=w255, error in=w259) -> (error out=w256:errorcluster)
      }
      frame "---------- UI ----------" {
        n65 = call <vilib>:"Add State(s) to Queue__JKI_lib_State_Machine.vi"("State(s) in (\"\")"=w264) -> ("States Out"=w263:string)  [unwired: 14 in]
      }
      frame "UI: Initialize" {
        n66 = call <vilib>:"Add State(s) to Queue__JKI_lib_State_Machine.vi"("State(s) in (\"\")"=w269) -> ("States Out"=w268:string)  [unwired: 14 in]
      }
      frame "UI: Cursor Set" {
        # "Argument"
        n67 = disable-structure shown="Default" {
          disable-tunnel: w273 -> [w279 w284]
          disable-tunnel: [w278 w284] -> w272
          disable-tunnel: w271 -> [w277 _]
          frame condition #0 (active) {
            n68 = case shown="\"Busy\"" w277 {
              tunnel: w279 -> [w281 w283]
              tunnel: [w280 w282] -> w278
              frame "Idle", Default {
                n69 = call <vilib>:"Unset Busy.vi"("error in (no error)"=w281) -> ("error out"=w280:errorcluster)  [unwired: 10 in]
              }
              frame "Busy" {
                n70 = call <vilib>:"Set Busy.vi"("error in (no error)"=w283) -> ("error out"=w282:errorcluster)  [unwired: 9 in, 1 out]
              }
            }
          }
          frame condition #1 {
          }
        }
        n71 = call <vilib>:"Add State(s) to Queue__JKI_lib_State_Machine.vi"("State(s) in (\"\")"=w276) -> ("States Out"=w275:string)  [unwired: 14 in]
      }
      frame "UI: Front Panel State" {
        # "Argument"
        n72 = Unbundle By Name(w288) -> ("Core.Current VI Reference"=w287:refnum<vi>)
        n73 = case shown="\"Minimize\", \"Minimized\"" w286 {
          tunnel: w290 -> [w298 w313 w324 w337 w350]
          tunnel: [w300 w314 w326 w339 w352] -> w289
          tunnel: w287 -> [w299 w311 w325 w338 w351]
          frame "Open", "Standard", Default {
            w293 = T1."Standard" ("State")
            n74 = property class="VI"(reference=w299, error in=w298) -> (reference out=w296:refnum<vi>, error out=w297:errorcluster, "FP.State"=w295:T1)
            n75 = Not Equal?(x=w295, y=w293) -> (x != y?=w294:bool)
            n76 = case shown="True" w294 {
              tunnel: [w304 w306] -> w300
              tunnel: w297 -> [w303 w306]
              tunnel: w296 -> [w302 _]
              tunnel: w293 -> [w301 _]
              frame True {
                n77 = invoke class="VI" method="FP.Open"(reference=w302, error in=w303, "Activate"=TRUE, "State"=w301) -> (error out=w304:errorcluster)  [unwired: 1 in, 4 out]
              }
              frame False {
              }
            }
          }
          frame "Close", "Closed" {
            n78 = property class="VI"(reference=w311, error in=w313) -> (reference out=w310:refnum<vi>, error out=w312:errorcluster, "FP.State"=w308:T1)
            n79 = Not Equal?(x=w308, y=T1."Closed" ("Front Panel Window:State")) -> (x != y?=w307:bool)
            n80 = case shown="True" w307 {
              tunnel: [w315 w318] -> w314
              tunnel: w312 -> [w315 w317]
              tunnel: w310 -> [_ w316]
              frame False {
              }
              frame True {
                n81 = invoke class="VI" method="FP.Close"(reference=w316, error in=w317) -> (error out=w318:errorcluster)  [unwired: 1 in, 2 out]
              }
            }
          }
          frame "Hidden", "Hide" {
            w319 = T1."Hidden" ("State")
            n82 = property class="VI"(reference=w325, error in=w324) -> (reference out=w322:refnum<vi>, error out=w323:errorcluster, "FP.State"=w321:T1)
            n83 = Not Equal?(x=w321, y=w319) -> (x != y?=w320:bool)
            n84 = case shown="True" w320 {
              tunnel: [w330 w331] -> w326
              tunnel: w323 -> [w329 w331]
              tunnel: w322 -> [w328 _]
              tunnel: w319 -> [w327 _]
              frame True {
                n85 = invoke class="VI" method="FP.Open"(reference=w328, error in=w329, "State"=w327) -> (error out=w330:errorcluster)  [unwired: 2 in, 4 out]
              }
              frame False {
              }
            }
          }
          frame "Minimize", "Minimized" {
            w332 = T1."Minimized" ("State")
            n86 = property class="VI"(reference=w338, error in=w337) -> (reference out=w335:refnum<vi>, error out=w336:errorcluster, "FP.State"=w334:T1)
            n87 = Not Equal?(x=w334, y=w332) -> (x != y?=w333:bool)
            n88 = case shown="False" w333 {
              tunnel: [w343 w344] -> w339
              tunnel: w336 -> [w342 w344]
              tunnel: w335 -> [w341 _]
              tunnel: w332 -> [w340 _]
              frame True {
                n89 = invoke class="VI" method="FP.Open"(reference=w341, error in=w342, "State"=w340) -> (error out=w343:errorcluster)  [unwired: 2 in, 4 out]
              }
              frame False {
              }
            }
          }
          frame "Maximize", "Maximized" {
            w345 = T1."Maximized" ("State")
            n90 = property class="VI"(reference=w351, error in=w350) -> (reference out=w348:refnum<vi>, error out=w349:errorcluster, "FP.State"=w347:T1)
            n91 = Not Equal?(x=w347, y=w345) -> (x != y?=w346:bool)
            n92 = case shown="True" w346 {
              tunnel: [w356 w357] -> w352
              tunnel: w349 -> [w355 w357]
              tunnel: w348 -> [w354 _]
              tunnel: w345 -> [w353 _]
              frame True {
                n93 = invoke class="VI" method="FP.Open"(reference=w354, error in=w355, "State"=w353) -> (error out=w356:errorcluster)  [unwired: 2 in, 4 out]
              }
              frame False {
              }
            }
          }
        }
        n94 = call <vilib>:"Add State(s) to Queue__JKI_lib_State_Machine.vi"("State(s) in (\"\")"=w292) -> ("States Out"=w291:string)  [unwired: 14 in]
      }
      frame "---------- Macro ----------" {
        n95 = call <vilib>:"Add State(s) to Queue__JKI_lib_State_Machine.vi"("State(s) in (\"\")"=w362) -> ("States Out"=w361:string)  [unwired: 14 in]
      }
      frame "Macro: Initialize" {
        w364 = "Data: Initialize\nInitialize Core Data\nEvents: Register\nUI: Initialize\nUI: Front Panel State >> Open"  # Data: Initialize Initialize Core Data Events: Register UI: Initialize UI: Front Panel State >> Open
        n96 = call <vilib>:"Add State(s) to Queue__JKI_lib_State_Machine.vi"("State(s) in Front (\"\")"=w364, "State(s) in (\"\")"=w368) -> ("States Out"=w367:string)  [unwired: 13 in]
      }
      frame "Macro: Exit" {
        n97 = Unbundle By Name(w376) -> ("Core.Close Panel on Exit?"=w375:bool)
        n98 = Select(t="UI: Front Panel State >> Close", s=w375, f="") -> (s? t:f=w372:string)
        n99 = call <vilib>:"Add State(s) to Queue__JKI_lib_State_Machine.vi"("State(s) in (\"\")"=w372, "State(s) at Back (\"\")"="Data: Cleanup\nEvents: Unregister\nExit") -> ("States Out"=w370:string)  [unwired: 13 in]
        n100 = call <vilib>:"Add State(s) to Queue__JKI_lib_State_Machine.vi"("State(s) in Front (\"\")"=w370, "State(s) in (\"\")"=w379) -> ("States Out"=w378:string)  [unwired: 13 in]
      }
      frame "---------- API ----------" {
      }
      frame "API: TestAPI" {
        w392 = T6 {"string"="xx", "bool"=FALSE, "dbl"=0.0, "cluster"={"string2"="zz", "bool2"=TRUE}}  # Arguments' Default Value
        # "Example for showing how to use CSM-API-String-Arugments-Support to simplify arguments input."
        # "#NOTE\nYou can change specified element's value with name:value pairs.\nDefault value will be used for unmentioned elements.\n\nFor example:\n\nArguments  = \"string:yy;cluster.bool2:Off;dbl:1M\" \n\nvalue of indicators should be:\n\nstring = yy\nbool = false\ndbl = 1,000,000\ncluster.string2 = zz\ncluster.bool2 = false"
        n101 = call "Convert API String Arguments to Data.vim"("Reference Type"=w392, "API String"=w391) -> ("error out"=w384:errorcluster, "Data"=w390:T6)  [unwired: 6 in]
        n102 = Unbundle By Name(w390) -> ("string"=→"string":string, "bool"=→"bool":bool, "dbl"=→"dbl":dbl, "cluster.string2"=→"cluster.string2":string, "cluster.bool2"=→"cluster.bool2":bool)
      }
      frame "API: API2" {
      }
      frame "---------- DoSth ----------" {
        n103 = call <vilib>:"Add State(s) to Queue__JKI_lib_State_Machine.vi"("State(s) in (\"\")"=w404) -> ("States Out"=w403:string)  [unwired: 14 in]
      }
      frame "DoSth: DoA" {
        n104 = call <vilib>:"Add State(s) to Queue__JKI_lib_State_Machine.vi"("State(s) in (\"\")"=w409) -> ("States Out"=w408:string)  [unwired: 14 in]
      }
      frame "DoSth: DoB" {
        n105 = call <vilib>:"Add State(s) to Queue__JKI_lib_State_Machine.vi"("State(s) in (\"\")"=w414) -> ("States Out"=w413:string)  [unwired: 14 in]
      }
    }
  }
  n106 = call "CSM - Query Internal Data Names By API String.vi"("Error In (no error)"=w10, "Target Module"=w5) -> ("error out"=w9:errorcluster, "Configurations"=→"Configurations":string[])  [unwired: 8 in]
  n107 = call <userlib>:"CSM - Send Message and Wait for Reply.vi"("Error In (No Error)"=w9, "Target Module"=w5, "Arguments (\"\")"="DataBool" ("Name(\"\" to use uuid)"), "State"=w22) -> ("error out"=w37:errorcluster, "Response"=→"DataBool":string)  [unwired: 5 in, 1 out]
  n108 = call <userlib>:"CSM - Send Message and Wait for Reply.vi"("Error In (No Error)"=w37, "Target Module"=w5, "Arguments (\"\")"="DataString" ("Name(\"\" to use uuid)"), "State"=w22) -> ("error out"=w35:errorcluster, "Response"=→"DataString":string)  [unwired: 5 in, 1 out]
  n109 = call <userlib>:"CSM - Send Message and Wait for Reply.vi"("Error In (No Error)"=w35, "Target Module"=w5, "Arguments (\"\")"="Settings.Bool" ("Name(\"\" to use uuid)"), "State"=w22) -> ("error out"=w36:errorcluster, "Response"=→"Settings.Bool":string)  [unwired: 5 in, 1 out]
  n110 = call <userlib>:"CSM - Send Message and Wait for Reply.vi"("Error In (No Error)"=w36, "Target Module"=w5, "Arguments (\"\")"="Settings.String" ("Name(\"\" to use uuid)"), "State"=w22) -> ("error out"=w24:errorcluster, "Response"=→"Settings.String":string)  [unwired: 5 in, 1 out]
  n111 = call <userlib>:"CSM - Send Message and Wait for Reply.vi"("Error In (No Error)"=w24, "Target Module"=w5, "Arguments (\"\")"="Settings" ("Name(\"\" to use uuid)"), "State"=w22) -> ("error out"=w19:errorcluster, "Response"=→"Settings":string)  [unwired: 5 in, 1 out]
  n112 = call <userlib>:"CSM - Send Message and Wait for Reply.vi"("Error In (No Error)"=w19, "Target Module"=w5, "Arguments (\"\")"="Core.Current VI Reference" ("Name(\"\" to use uuid)"), "State"="Data: Get Internal Data" ("Name(\"\" to use uuid)")) -> ("error out"=w14:errorcluster, "Response"=w16:string)  [unwired: 5 in, 1 out]
  "Core.Current VI Reference" <- w16
  n113 = call <userlib>:"CSM - Module VI Reference.vi"("error in (no error)"=w14, "CSM Name"=w5) -> ("error out"=w13:errorcluster, "CSM Module VIRef"=w12:refnum<vi>)  [unwired: 8 in]
  n114 = property class="VI"(reference=w12) -> ("Path"=→"VI Path":path)  [unwired: 1 in, 2 out]
  n115 = flat-sequence {
    tunnel: [w416] -> w20
    tunnel: w13 -> [w416]
    frame #0 {
      n116 = Wait (ms)(milliseconds to wait=u32 1000) -> ()  [unwired: 1 out]
    }
  }
  n117 = call <userlib>:"CSM - Convert HexStr to Data.vi"("HEX String"=w16) -> ("Variant"=→"Core.Current VI Reference":variant)  [unwired: 7 in, 1 out]
  n118 = disable-structure shown="Enabled" {
    disable-tunnel: w20 -> [w420 w421]
    disable-tunnel: [w419 w421] -> w26
    disable-tunnel: "Macro: Exit" ("Name(\"\" to use uuid)") -> [w418 _]
    disable-tunnel: w5 -> [w417 _]
    frame Enabled {
      n119 = call <userlib>:"CSM - Send Message and Wait for Reply.vi"("Error In (No Error)"=w420, "Target Module"=w417, "State"=w418) -> ("error out"=w419:errorcluster)  [unwired: 6 in, 2 out]
    }
    frame Disabled {
    }
  }
  "error out" <- w26
